vi "As YX Projection.vi"(11 "Hailstone in":refnum<class "Hailstone.lvclass">) -> (2 "Trace":refnum<class "Trace.lvclass">)   [LabVIEW 2021]
uses:
  Hailstone.lvclass/Hailstone.ctl
  Trace/Trace.lvclass
  High Res Arithmetic/High Res Arithmetic.lvclass
  Hailstone.lvclass
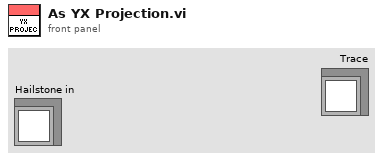
[diagram p1: front panel]
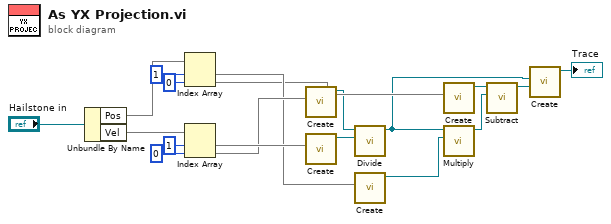
[diagram p0: block diagram]
diagram:
  n1 = Unbundle By Name("Hailstone in") -> ("Pos"=w19, "Vel"=w16)
  n2 = Index Array(array=w19, index #1=1 ("index"), index #2=0 ("index")) -> (element #1=w12, element #2=w10)
  n3 = Index Array(array=w16, index #1=1 ("index"), index #2=0 ("index")) -> (element #1=w15, element #2=w14)
  n4 = call "Create.vi"("Numerator"=w14) -> ("Hi Res Arithm Test"=w6:refnum<class "High Res Arithmetic.lvclass">)  [unwired: 9 in, 1 out]
  n5 = call "Create.vi"("Numerator"=w15) -> ("Hi Res Arithm Test"=w13:refnum<class "High Res Arithmetic.lvclass">)  [unwired: 9 in, 1 out]
  n6 = call "Divide.vi"("High Res Arithmetic 2"=w13, "High Res Arithmetic 1"=w6) -> ("High Res Arithmetic sum"=w5:refnum<class "High Res Arithmetic.lvclass">)  [unwired: 8 in, 1 out]
  n7 = call "Create.vi"("Numerator"=w12) -> ("Hi Res Arithm Test"=w11:refnum<class "High Res Arithmetic.lvclass">)  [unwired: 9 in, 1 out]
  n8 = call "Create.vi"("Numerator"=w10) -> ("Hi Res Arithm Test"=w9:refnum<class "High Res Arithmetic.lvclass">)  [unwired: 9 in, 1 out]
  n9 = call "Multiply.vi"("High Res Arithmetic 2"=w11, "High Res Arithmetic 1"=w5) -> ("High Res Arithmetic sum"=w8:refnum<class "High Res Arithmetic.lvclass">)  [unwired: 8 in, 1 out]
  n10 = call "Subtract.vi"("High Res Arithmetic 2"=w8, "High Res Arithmetic 1"=w9) -> ("High Res Arithmetic sum"=w7:refnum<class "High Res Arithmetic.lvclass">)  [unwired: 8 in, 1 out]
  n11 = call "Create.vi"("Offset"=w7, "Slope"=w5) -> ("Trace"=→"Trace":refnum<class "Trace.lvclass">)  [unwired: 8 in, 1 out]
